vi "SetProcessSyncRendezvousSize.vi"(8 "error in":errorcluster, 10 "# processes":i32, 11 "Process Sync Rendezvous":T1) -> (0 "error out":errorcluster)   [LabVIEW 2013, in "SMO.lvclass"]
doc: "Sets the size of the Process Sync Rendezvous in the JKI SMO.\n\n---------------------------------------------------------------\nJKI State Machine Objects™\nhttp://jki.net/state-machine-objects/\nCopyright (C) 2005-2015, JKI <info@jki.net>\nALL RIGHTS RESERVED"
uses:
  SMO.lvclass
panel:
  # "For instructions on how to use the JKI State Machine Objects, examples and video tutorials, visit:\nhttp://jki.net/state-machine-objects/\n\nJKI State Machine Objects™\nhttp://jki.net/state-machine-objects/\nCopyright (C) 2005-2015, JKI <info@jki.net>\nALL RIGHTS RESERVED"
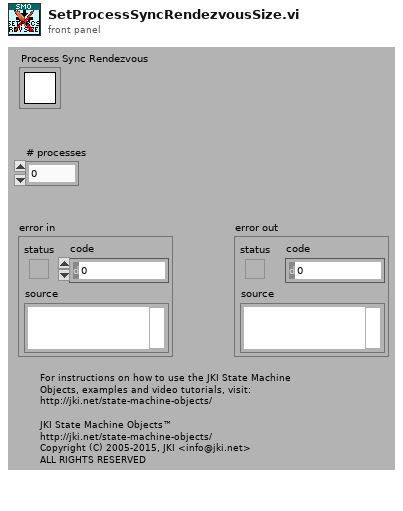
[diagram p1: front panel]
types:
  T1 = typedef "Rendezvous RefNum" = refnum<k1>
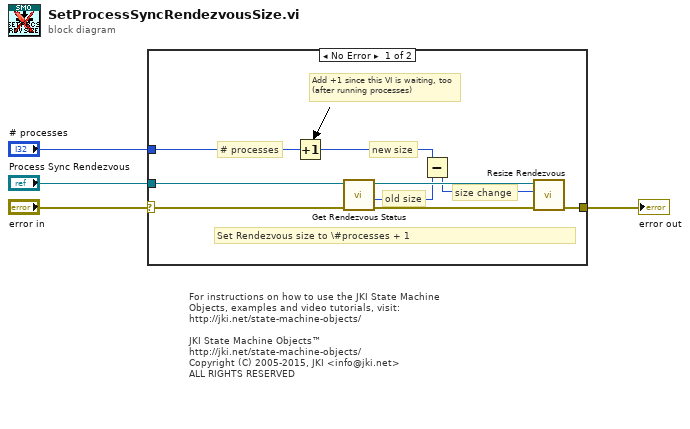
[diagram p0: block diagram]
diagram:
  # "For instructions on how to use the JKI State Machine Objects, examples and video tutorials, visit:\nhttp://jki.net/state-machine-objects/\n\nJKI State Machine Objects™\nhttp://jki.net/state-machine-objects/\nCopyright (C) 2005-2015, JKI <info@jki.net>\nALL RIGHTS RESERVED"
  n1 = case shown="No Error" "error in" {
    selector: "error in" -> [w6 w14]
    tunnel: "Process Sync Rendezvous" -> [w13 _]
    tunnel: [w7 w14] -> w3
    tunnel: "# processes" -> [w5 _]
    frame No Error {
      # "Set Rendezvous size to \\#processes + 1"
      # "Add +1 since this VI is waiting, too (after running processes)"
      # "# processes"
      # "size change"
      # "new size"
      # "old size"
      n2 = Increment(x=w5) -> (x+1=w12:i32)
      n3 = call <vilib>:"Get Rendezvous Status.vi"("error in (no error)"=w6, "rendezvous"=w13) -> ("error out"=w10:errorcluster, "size"=w9:i32, "rendezvous out"=w11:T1)  [unwired: 7 out]
      n4 = Subtract(x=w12, y=w9) -> (x-y=w8:i32)
      n5 = call <vilib>:"Resize Rendezvous.vi"("error in (no error)"=w10, "size change (0)"=w8, "rendezvous"=w11) -> ("error out"=w7:errorcluster)  [unwired: 4 out]
    }
    frame Error {
    }
  }
  "error out" <- w3
